vi "booleanos.vi"() -> ()   [LabVIEW 2020]
panel:
  in  "Boton 2":bool
  in  "Boton1":bool
  # "Booleanos"
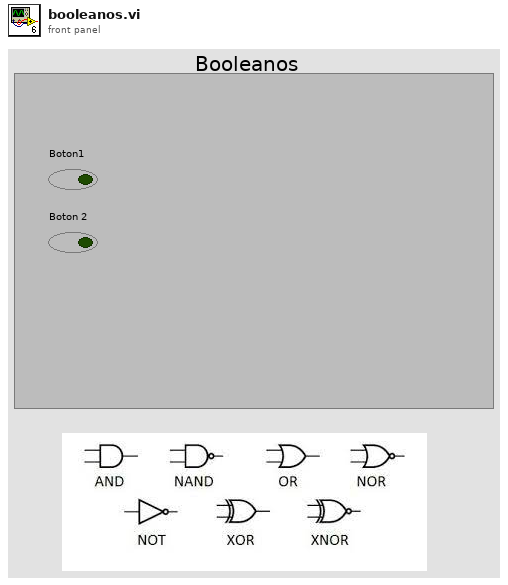
[diagram p1: front panel]
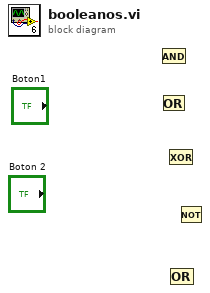
[diagram p0: block diagram]
diagram:
  n1 = And() -> ()  [unwired: 2 in, 1 out]
  n2 = Or() -> ()  [unwired: 2 in, 1 out]
  n3 = Exclusive Or() -> ()  [unwired: 2 in, 1 out]
  n4 = Compound Arithmetic op=OR() -> ()  [unwired: 2 in, 1 out]
  n5 = Not() -> ()  [unwired: 1 in, 1 out]
